vi "DUAL GAUGE-Test Memory.vi"(8 "Fehler (Eingang)":errorcluster, 9 "Testfunction":u8(ring) items=["EEPROM Test", "EPROM Test", "RAM Test"], 11 "Referenz in":refnum<visa-resource-name>) -> (0 "Cluster (Ausgang)":errorcluster, 1 "Errortext":string, 2 "Errornumber":u16, 3 "Referenz out":refnum<visa-resource-name>)   [LabVIEW 2010, in "Dual Gauge.lvlib"]
uses:
  Dual Gauge.lvlib
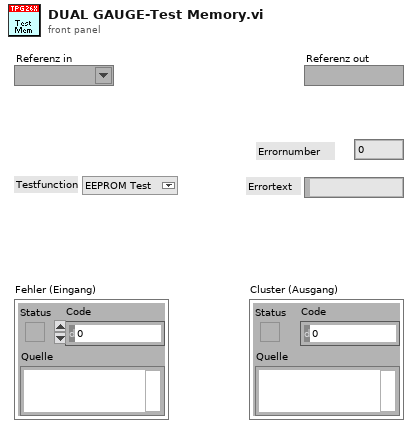
[diagram p1: front panel]
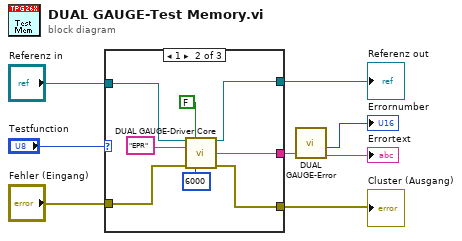
[diagram p0: block diagram]
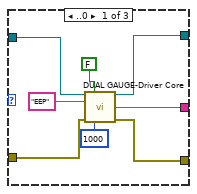
[diagram p2: hidden frame]
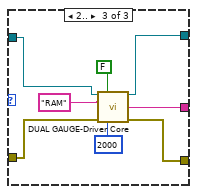
[diagram p3: hidden frame]
diagram:
  n1 = case shown="1" "Testfunction" {
    tunnel: [w16 w22 w30] -> w5
    tunnel: [w13 w23 w31] -> w4
    tunnel: "Fehler (Eingang)" -> [w11 w17 w25]
    tunnel: "Referenz in" -> [w10 w19 w27]
    tunnel: [w9 w18 w26] -> w1
    frame ..0 {
      n2 = call "DUAL GAUGE-Driver Core.vi"("Referenz in"=w10, "Write/Read"=FALSE, "Command"="EEP", "Fehler (Eingang)"=w11, "Timeout [ms]"=u32 1000) -> ("Referenz out"=w9:refnum<visa-resource-name>, "String Out"=w16:string, "Cluster (Ausgang)"=w13:errorcluster)  [unwired: 8 in]
    }
    frame 1 {
      n3 = call "DUAL GAUGE-Driver Core.vi"("Referenz in"=w19, "Write/Read"=FALSE, "Command"="EPR", "Fehler (Eingang)"=w17, "Timeout [ms]"=u32 6000) -> ("Referenz out"=w18:refnum<visa-resource-name>, "String Out"=w22:string, "Cluster (Ausgang)"=w23:errorcluster)  [unwired: 8 in]
    }
    frame 2.. {
      n4 = call "DUAL GAUGE-Driver Core.vi"("Referenz in"=w27, "Write/Read"=FALSE, "Command"="RAM", "Fehler (Eingang)"=w25, "Timeout [ms]"=u32 2000) -> ("Referenz out"=w26:refnum<visa-resource-name>, "String Out"=w30:string, "Cluster (Ausgang)"=w31:errorcluster)  [unwired: 8 in]
    }
  }
  "Cluster (Ausgang)" <- w4
  "Referenz out" <- w1
  n5 = call "DUAL GAUGE-Error.vi"("String IN"=w5) -> ("Errortext"=→"Errortext":string, "Errornumber"=→"Errornumber":i32)  [unwired: 8 in]
